vi "Read Hardware.lvlib_CCD.lvlib_CCD.lvclass.vi"(8 "error in (no error)":errorcluster, 11 "CCD Configuration in":refnum<class "CCD Configuration.lvclass">) -> (0 "error out":errorcluster, 2 "Hardware.lvlib:CCD.lvlib:CCD.lvclass":refnum<class "CCD.lvclass">, 3 "CCD Configuration out":refnum<class "CCD Configuration.lvclass">)   [LabVIEW 2016, in "CCD.lvlib" / "CCD Configuration.lvclass"]
uses:
  <userlib>/Common Components/Hardware/CCD/CCD Configuration.lvclass
  <userlib>/Common Components/Hardware/CCD/CCD/CCD.lvclass
  <userlib>/Common Components/Hardware/CCD/CCD Configuration.lvclass/CCD Configuration.ctl
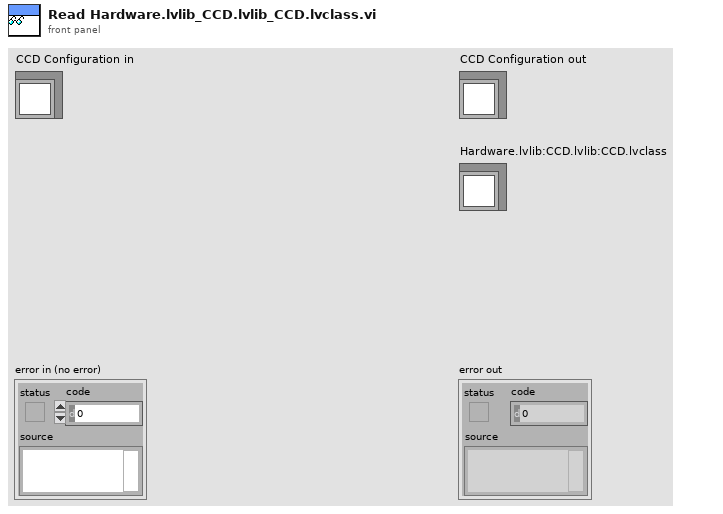
[diagram p1: front panel]
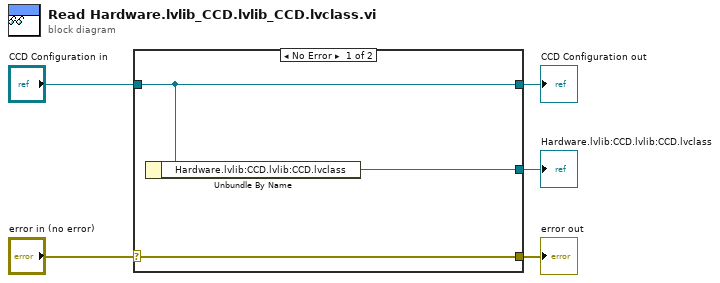
[diagram p0: block diagram]
diagram:
  n1 = case shown="No Error" "error in (no error)" {
    selector: "error in (no error)" -> [w8 w9]
    tunnel: [w8 w9] -> w4
    tunnel: [w7 w10] -> w2
    tunnel: "CCD Configuration in" -> [w7 w10]
    tunnel: [w6 _] -> w1
    frame No Error {
      n2 = Unbundle By Name(w7) -> ("Hardware.lvlib:CCD.lvlib:CCD.lvclass"=w6:refnum<class "CCD.lvclass">)
    }
    frame Error {
    }
  }
  "error out" <- w4
  "CCD Configuration out" <- w2
  "Hardware.lvlib:CCD.lvlib:CCD.lvclass" <- w1
